vi "CD Pth Type To Absolute.vi"(8 "error in (no error)":errorcluster, 11 "CD Path Pair":T1) -> (0 "error out":errorcluster, 3 "Absolute Path":path)   [LabVIEW 2026, in "Custom Devices Storage.lvlib"]
uses:
  Custom Devices Storage.lvlib
  <vilib>/NI VeriStand/Custom Device API/Path Type.ctl
  <vilib>/NI VeriStand/Custom Device API/Custom Device API.lvlib
  <vilib>/NI VeriStand/Custom Device API/Path Specification.ctl
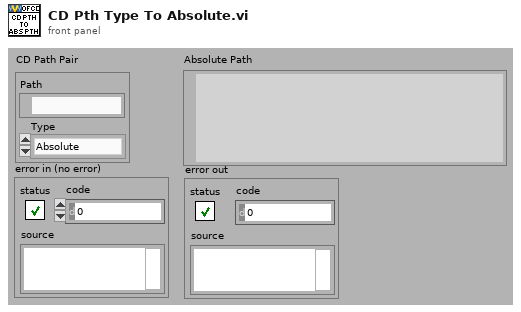
[diagram p1: front panel]
types:
  T1 = typedef "Custom Device API.lvlib/Path Specification.ctl" = cluster{"Path":path, "Type":T2}
  T2 = typedef "Custom Device API.lvlib/Path Type.ctl" = enum16{"Absolute", "To Base", "To Common Data Dir", "To Application Data Dir"}
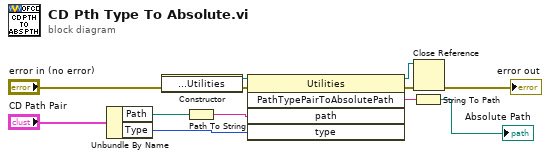
[diagram p0: block diagram]
diagram:
  n1 = Unbundle By Name("CD Path Pair") -> ("Path"=w5:path, "Type"=w3:T2)
  n2 = constructor class="Utilities"(error in="error in (no error)") -> (reference out=w12:refnum<k39>, error out=w11:errorcluster)  [unwired: 2 in, 1 out]
  n3 = Path To String(path=w5) -> (string=w4:string)
  n4 = invoke class="Utilities" method="PathTypePairToAbsolutePath"(reference=w12, error in=w11, "path"=w4, "type"=w3) -> (reference out=w8:refnum<k39>, error out=w9:errorcluster, "PathTypePairToAbsolutePath"=w2:string)  [unwired: 1 in, 2 out]
  n5 = String To Path(string=w2) -> (path=→"Absolute Path":path)
  n6 = Close Reference(reference=w8, error in (no error)=w9) -> (error out=→"error out":errorcluster)
